vi "Catch Nested Value Update.vi"(8 "error in (no error)":errorcluster, 10 "Nested Value Update Msg":refnum<class "Nested Value Update Msg.lvclass">, 11 "TopLevelApplication In":refnum<class "ConcreteViewModel.lvclass">) -> (0 "error out":errorcluster, 3 "TopLevelApplication Out":refnum<class "ConcreteViewModel.lvclass">)   [LabVIEW 2017, in "Integration Test Launcher.lvlib" / "TopLevelApplication.lvlib" / "ConcreteViewModel.lvclass"]
doc: "<License>\nCopyright © 2020 Tymphany, LLC | All rights reserved\nwww.Tymphany.com\nHuijun <Huijun.Guo@Tymphany.com>\n</License>"
uses:
  <vilib>/gpm_packages/@cs/example/Integration Test/ConcreteViewModel/ConcreteViewModel.lvclass
  <vilib>/gpm_packages/@cs/mva-viewable/Source/IViewable/IViewable Messages/Catch Nested Value Change Msg/Nested Value Update Msg.lvclass
  <vilib>/gpm_packages/@cs/mva-viewable/Source/IViewable/IViewable Messages/Catch Nested Value Change Msg/Nested Value Update Msg.lvclass/Nested Value Update Msg.ctl
  <vilib>/Utility/Data Type/NI_Data Type.lvlib
  <vilib>/gpm_packages/@cs/mva-dialogbox/source/OneButtonDialogBox/OneButtonDialogBox.lvclass
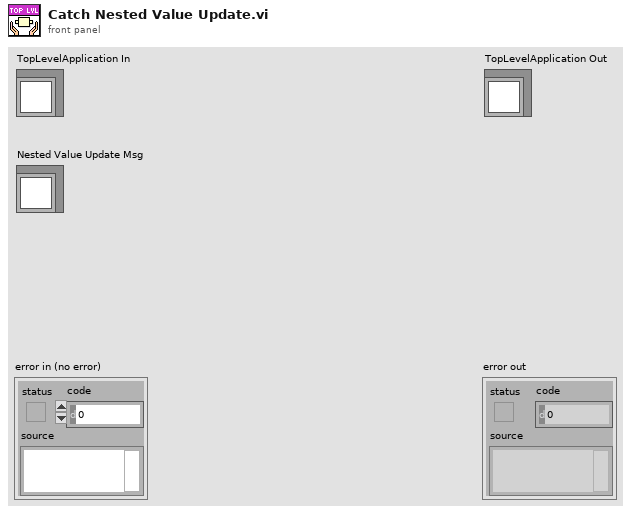
[diagram p1: front panel]
types:
  T1 = typedef "NI_Data Type.lvlib/Data Type.ctl" = enum8{"Invalid Type", "Void", "I8", "I16", "I32", "I64", "U8", "U16", "U32", "U64", "Single Float", "Double Float", "Extended Float", "Single Complex", "Double Complex", "Extended Complex", "Enum U8", "Enum U16", "Enum U32", "Enum U64", "Single Float With Unit", "Double Float With Unit", "Extended Float With Unit", "Single Complex with Unit", "Double Complex with Unit", "Extended Complex with Unit", "Boolean", "String", "Path", "Picture", "Tag", "Array", "Cluster", "Variant", "LV Variant", "Waveform", "Timestamp", "Digital Waveform", "Digital Data", "ExpressData", "Refnum", "External Data", "VI", "Poly VI", "LabVIEW Class Instance", "Fixed Point"}
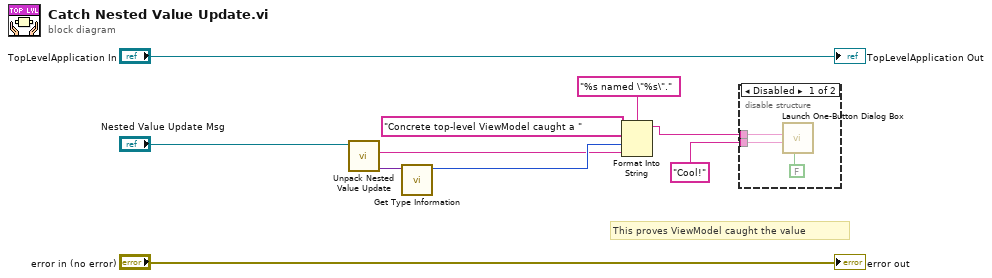
[diagram p0: block diagram]
diagram:
  # "This proves ViewModel caught the value"
  n1 = call <vilib>:"Unpack Nested Value Update.vi"("Nested Value Update Msg"="Nested Value Update Msg") -> ("Value"=w5:variant, "Datum Name"=w4:string)  [unwired: 8 in, 1 out]
  n2 = call <vilib>:"Get Type Information.vi"("Variant"=w5) -> ("Type"=w6:T1)  [unwired: 6 in, 4 out]
  n3 = Format Into String(format string="%s named \"%s\".", initial string="Concrete top-level ViewModel caught a ", w6, w4) -> (resulting string=w1:string)  [unwired: 1 in, 1 out]
  n4 = disable-structure shown="Disabled" {
    disable-tunnel: "Cool!" ("Button Text (OK)") -> [w13 _]
    disable-tunnel: w1 -> [w12 _]
    frame Disabled {
      n5 = call <vilib>:"Launch One-Button Dialog Box.vi"("Modal? (T)"=FALSE, "Button Text (OK)"=w13, "Message Text"=w12) -> ()  [unwired: 8 in, 1 out]
    }
    frame Enabled {
    }
  }
  "error out" <- "error in (no error)"
  "TopLevelApplication Out" <- "TopLevelApplication In"
